vi "DigitalWaveformProbe.vi"(1 "Digital Waveform":digitalwaveform(waveform)) -> (0 "Stop if?":bool)   [LabVIEW 2017]
doc: "Displays a graph of the digital data; a table with a time stamp that specifies when the probe received the data, the x value, and the time; and a table that displays the attributes of the waveform data type."
panel:
  in  "Tab Control":T1(tab)
  out "Timestamp":timestamp format="%<%X\n%x>T"
  out "Digital Waveform Graph":digitalwaveform(graph)
  out "dt":dbl format="%.6f"
  out "t0":timestamp format="%<%X\n%x>T"
  out "Y":digitaldata
  out "Attributes":variant
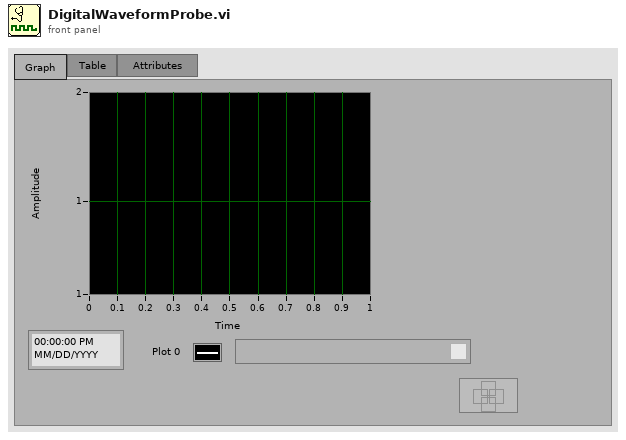
[diagram p1: front panel]
types:
  T1 = enum32{"Graph   ", "Table   ", "Attributes      "}
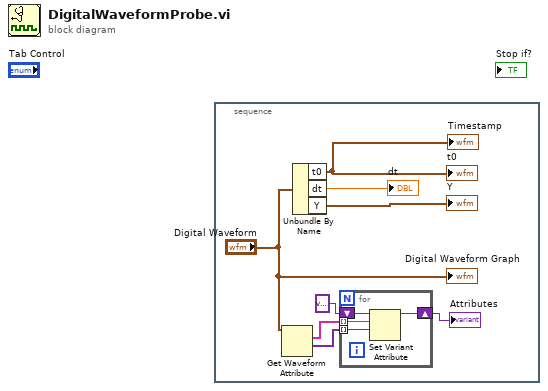
[diagram p0: block diagram]
diagram:
  n1 = stacked-sequence {
    frame #0 {
      n2 = Get Waveform Attribute(7:"Digital Waveform") -> (1:w3:variant[], 2:w4:string[])  [unwired: 3 in, 2 out]
      n3 = Unbundle By Name("Digital Waveform") -> ("t0"=→"Timestamp" →"t0":timestamp, "dt"=→"dt":dbl, "Y"=→"Y":digitaldata)
      n4 = for {
        tunnel: w4 -> [w12] mode=indexing
        tunnel: w3 -> [w11] mode=indexing
        shift-right: [w9] -> w1
        shift-left: variant ("variant") -> [w10]
        n5 = Set Variant Attribute(Variant=w10, name=w12, value=w11) -> (Variant out=w9:variant)  [unwired: 1 in, 2 out]
      }
      "Attributes" <- w1
      "Digital Waveform Graph" <- "Digital Waveform"
    }
  }
